vi "element_editor_list_hydrolyse.vi"(11 "path":path) -> (0 "path to folder":path, 1 "indexes":string[](array[string]), 2 "full_names":string[](array[string]), 3 "Value":string)   [LabVIEW 2019]
panel:
  in  "Button":bool
  in  "Reactors":string(combo)
  # "Choose the reactor:"
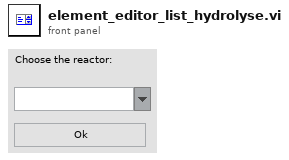
[diagram p1: front panel]
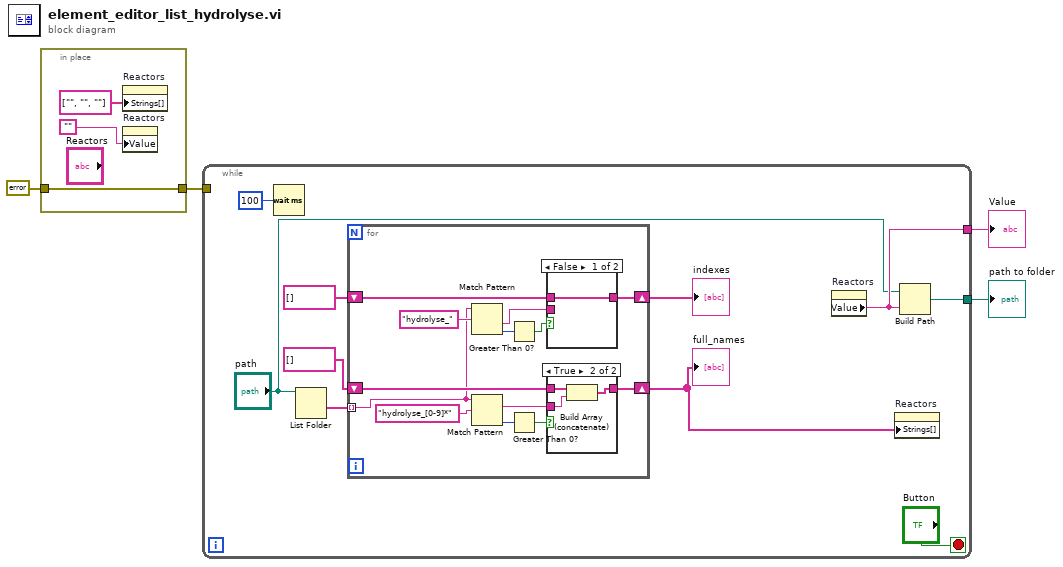
[diagram p0: block diagram]
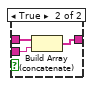
[diagram p2: hidden frame]
diagram:
  n1 = in-place {
    in-place-border: errorcluster {"status"=FALSE, "code"=0, "source"=""} ("error constant") -> [w6]
    in-place-border: [w6] -> w1
    n2 = property on="Reactors" class="CmbBox"("Strings[]"=string[] ["", "", ""] ("full_names")) -> ()  [unwired: 2 in, 2 out]
    n3 = property on="Reactors" class="CmbBox"("Value"="") -> ()  [unwired: 2 in, 2 out]
  }
  n4 = while {
    tunnel: [w11] -> w4
    tunnel: [w9] -> w3
    tunnel: w1 -> [_]
    stop <- "Button" stop-if-true
    n5 = Wait (ms)(milliseconds to wait=u32 100) -> ()  [unwired: 1 out]
    n6 = List Folder(path="path") -> (folder names=w17:string[])  [unwired: 3 in, 3 out]
    n7 = for {
      tunnel: w17 -> [w18] mode=indexing
      shift-right: [w25] -> w8
      shift-left: string[] [] -> [w27]
      shift-right: [w21] -> w14
      shift-left: string[] [] ("Array") -> [w20]
      n8 = Match Pattern(string=w18, regular expression="hydrolyse_" ("string")) -> (after substring=w22:string, offset past match=w24:i32)  [unwired: 1 in, 2 out]
      n9 = Match Pattern(string=w18, regular expression="hydrolyse_[0-9]*") -> (match substring=w26:string, offset past match=w28:i32)  [unwired: 1 in, 2 out]
      n10 = Greater Than 0?(x=w24) -> (x > 0?=w23:bool)
      n11 = Greater Than 0?(x=w28) -> (x > 0?=w29:bool)
      n12 = case shown="False" w23 {
        tunnel: w22 -> [_ w34]
        tunnel: [w31 w33] -> w21
        tunnel: w20 -> [w31 w32]
        frame False {
        }
        frame True {
          n13 = Build Array (concatenate)(w32, w34) -> (w33:string[])
        }
      }
      n14 = case shown="True" w29 {
        tunnel: [w35 w38] -> w25
        tunnel: w27 -> [w35 w37]
        tunnel: w26 -> [_ w36]
        frame False {
        }
        frame True {
          n15 = Build Array (concatenate)(w37, w36) -> (w38:string[])
        }
      }
    }
    "full_names" <- w8
    "indexes" <- w14
    n16 = property on="Reactors" class="CmbBox"() -> ("Value"=w11:string)  [unwired: 2 in, 2 out]
    n17 = property on="Reactors" class="CmbBox"("Strings[]"=w8) -> ()  [unwired: 2 in, 2 out]
    n18 = Build Path(base path="path", name or relative path=w11) -> (appended path=w9:path)
  }
  "Value" <- w4
  "path to folder" <- w3
